vi "1553 Debug Parser.vi"() -> ()   [LabVIEW 2016]
panel:
  in  "Bad File":bool
  out "Debug Data":string[][](array[string])
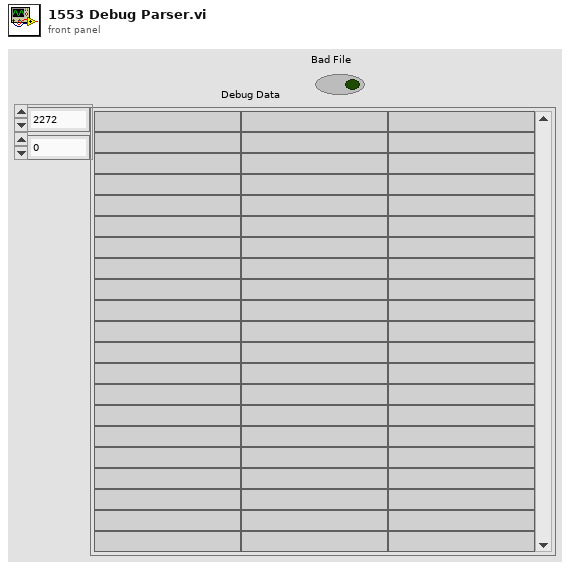
[diagram p1: front panel]
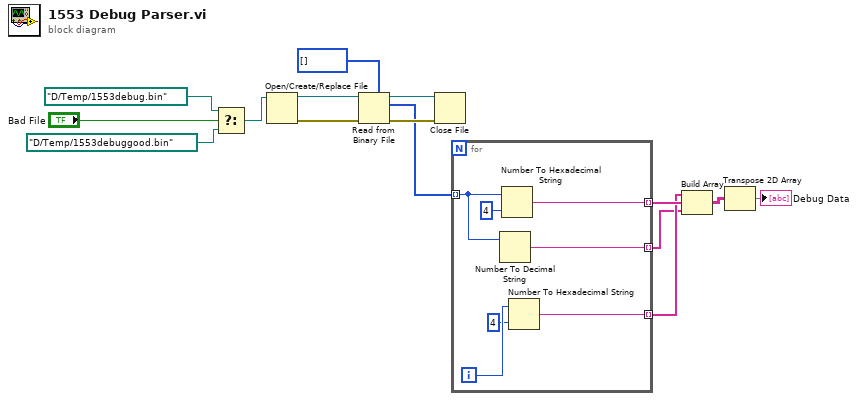
[diagram p0: block diagram]
diagram:
  n1 = Select(t=path "D:/Temp/1553debug.bin" ("file path (use dialog)"), s="Bad File", f=path "D:/Temp/1553debuggood.bin" ("file path (use dialog)")) -> (s? t:f=w4:path)
  n2 = Open/Create/Replace File(file path (use dialog)=w4) -> (refnum out=w15:refnum<file>, error out=w14:errorcluster)  [unwired: 5 in, 1 out]
  n3 = Read from Binary File(5:u16[] [], 8:w14, 11:w15) -> (0:w12:errorcluster, 2:w10:u16[], 3:w13:refnum<file>)  [unwired: 3 in, 1 out]
  n4 = Close File(refnum=w13, error in=w12) -> ()  [unwired: 2 out]
  n5 = for {
    tunnel: w10 -> [w17] mode=indexing
    tunnel: [w19] -> w8 mode=indexing
    tunnel: [w18] -> w9 mode=indexing
    tunnel: [w16] -> w1 mode=indexing
    i -> [w22]
    n6 = Number To Decimal String(number=w17) -> (decimal integer string=w16:string)  [unwired: 1 in]
    n7 = Number To Hexadecimal String(1:i16 4 ("width (-)"), 2:w17) -> (0:w18:string)
    n8 = Number To Hexadecimal String(1:i16 4 ("width (-)"), 2:w22) -> (0:w19:string)
  }
  n9 = Build Array(w8, w9, w1) -> (w7:string[][])
  n10 = Transpose 2D Array(2D array=w7) -> (transposed array=→"Debug Data":string[][])
